vi "RunProcess.vi"(8 "error in (no error)":errorcluster, 11 ".NET Process in":refnum<class "SystemProcessManager.lvclass">) -> (0 "error out":errorcluster, 3 ".NET Process out":refnum<class "SystemProcessManager.lvclass">)   [LabVIEW 2019, in "SystemProcessManager.lvclass"]
uses:
  SystemProcessManager.lvclass
  SystemProcessManager.lvclass/SystemProcessManager.ctl
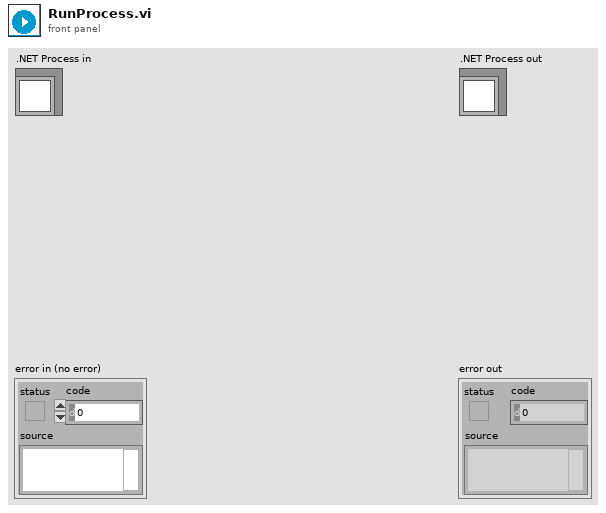
[diagram p1: front panel]
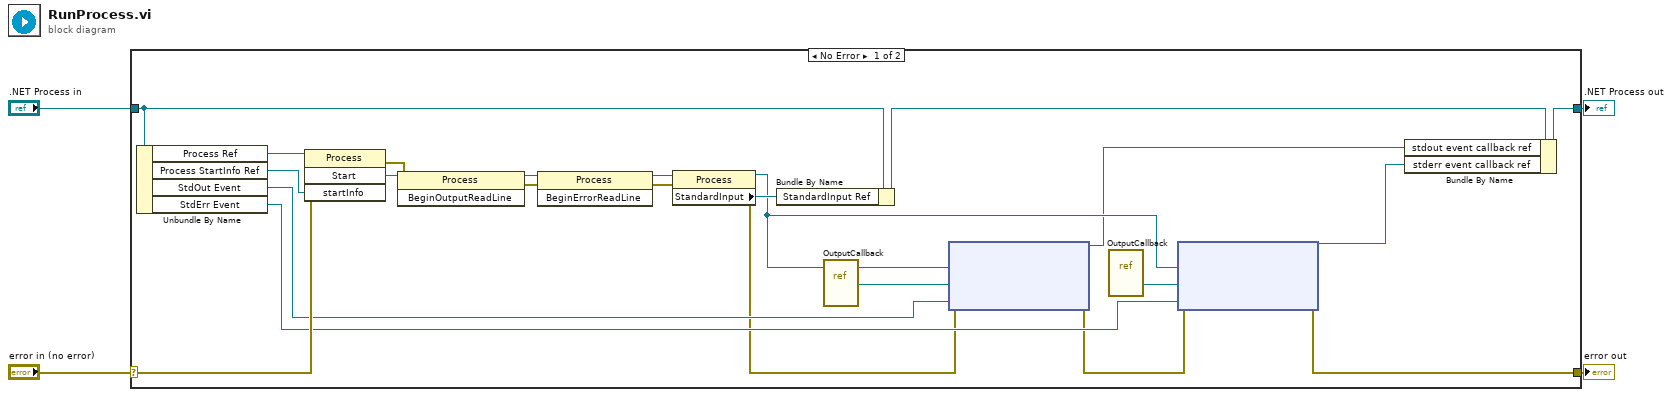
[diagram p0: block diagram]
diagram:
  n1 = case shown="No Error" "error in (no error)" {
    selector: "error in (no error)" -> [w19 w29]
    tunnel: [w10 w29] -> w3
    tunnel: [w7 w28] -> w1
    tunnel: ".NET Process in" -> [w18 w28]
    frame No Error {
      n2 = Unbundle By Name(w18) -> ("Process Ref"=w25:refnum<k24>, "Process StartInfo Ref"=w24:refnum<k24>, "StdOut Event"=w15:refnum<user-event>, "StdErr Event"=w14:refnum<user-event>)
      n3 = invoke class="Process" method="Start"(reference=w25, error in=w19, "startInfo"=w24) -> (error out=w23:errorcluster, "Start"=w22:refnum<k24>)  [unwired: 1 in, 2 out]
      n4 = invoke class="Process" method="BeginOutputReadLine"(reference=w22, error in=w23) -> (reference out=w27:refnum<k24>, error out=w26:errorcluster)  [unwired: 1 in, 1 out]
      n5 = invoke class="Process" method="BeginErrorReadLine"(reference=w27, error in=w26) -> (reference out=w21:refnum<k24>, error out=w20:errorcluster)  [unwired: 1 in, 1 out]
      n6 = property class="Process"(reference=w21, error in=w20) -> (reference out=w9:refnum<k24>, error out=w12:errorcluster, "StandardInput"=w17:refnum<k24>)
      n7 = Bundle By Name(cluster=w18, "StandardInput Ref"=w17) -> (w8:refnum<class "SystemProcessManager.lvclass">)
      n8 = vi-ref "OutputCallback.vi"() -> ("vi reference"=w16:refnum<vi>)
      n9 = node(w12, w9, w16, w15) -> (w6:refnum<k27>, w11:errorcluster)  [unwired: 1 in]
      n10 = vi-ref "OutputCallback.vi"() -> ("vi reference"=w13:refnum<vi>)
      n11 = node(w11, w9, w13, w14) -> (w5:refnum<k27>, w10:errorcluster)  [unwired: 1 in]
      n12 = Bundle By Name(cluster=w8, "stdout event callback ref"=w6, "stderr event callback ref"=w5) -> (w7:refnum<class "SystemProcessManager.lvclass">)
    }
    frame Error {
    }
  }
  "error out" <- w3
  ".NET Process out" <- w1
